vi "MeasureRMS.vi"(10 "# of Samples":dbl, 11 "Sampling Rate (Hz)":dbl) -> (1 "Waveform Graph":dbl[](graph), 2 "RMS":dbl)   [LabVIEW 2015]
uses:
  <vilib>/Analysis/NI_AALPro.lvlib
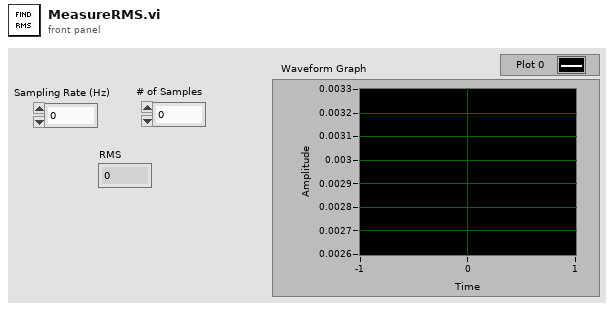
[diagram p1: front panel]
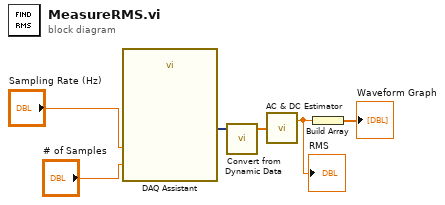
[diagram p0: block diagram]
diagram:
  n1 = call "DAQ Assistant"("rate"="Sampling Rate (Hz)", "number of samples"="# of Samples") -> ("data"=w6:dynamicdata)  [unwired: 15 in, 2 out]
  n2 = call "Convert from Dynamic Data"("Dynamic Data Type"=w6) -> ("Array"=w5:dbl[])  [unwired: 3 in]
  n3 = call <vilib>:"AC & DC Estimator.vi"("Signal (V)"=w5) -> ("AC estimate (Vrms)"=w2:dbl)  [unwired: 1 out]
  "RMS" <- w2
  n4 = Build Array(w2) -> (→"Waveform Graph":dbl[])
